vi "CS_schleife_init.vi"   [LabVIEW 2016]
uses:
  Global/Global Variables/global.vi
  Global/Global Variables/Data_Display_global.vi
  Instrument_Setup.vi
  Monitors/Utility/Monitor Communication/sub-vis/16T_Split_Cluster.vi
  Monitors/Utility/Monitor Communication/sub-vis/20T_Split_Cluster.vi
  Monitors/Utility/Monitor Communication/sub-vis/SR830_Open_Queue.vi
  Monitors/Utility/Monitor Communication/sub-vis/16T_Queue_Commands.vi
  Monitors/Utility/Monitor Communication/sub-vis/20T_Open_Queue.vi
  Monitors/Utility/Monitor Communication/sub-vis/20T_Queue_Commands.vi
types:
  T1 = typedef "16T-Cluster.ctl" = cluster{"Clamp":bool, "Switch Heater":bool, "Go to Zero":bool, "Go to set":bool, "Go to Hold":bool, "Clamped":bool, "Quenched":bool, "Rate limit":bool, "Persistent":bool, "Hold":bool, "Set":bool, "Zero":bool, "Magnet (T)":dbl, "Leads (T)":dbl, "Magnet T (K)":dbl, "Switch":bool, "Setpoint (T)":dbl, "Rate (T/min)":dbl, "Select":bool, "Sweeping":bool}
  T2 = typedef "16T_Control.ctl" = cluster{"Clamp":bool, "Switch Heater":bool, "Go to Zero":bool, "Go to Set":bool, "Go to Hold":bool, "Setpoint (T)":dbl, "Rate (T/min)":dbl, "Set Rate":bool}
  T3 = typedef "20T_Cluster.ctl" = cluster{"Clamp":bool, "Switch Heater":bool, "Go to Zero":bool, "Go to set":bool, "Go to Hold":bool, "Clamped":bool, "Quenched":bool, "Rate limit":bool, "Persistent":bool, "Hold":bool, "Set":bool, "Zero":bool, "Magnet (T)":dbl, "Leads (T)":dbl, "Magnet T (K)":dbl, "Switch":bool, "Target (T)":dbl, "Setpoint (T)":dbl, "Rate (T/min)":dbl, "Switch Heater 2":bool, "Set Rate":bool}
  T4 = typedef "20T_Control.ctl" = cluster{"Clamp":bool, "Switch Heater":bool, "Go to Zero":bool, "Go to Set":bool, "Go to Hold":bool, "Setpoint (T)":dbl, "Rate (T/min)":dbl, "Set Rate":bool}
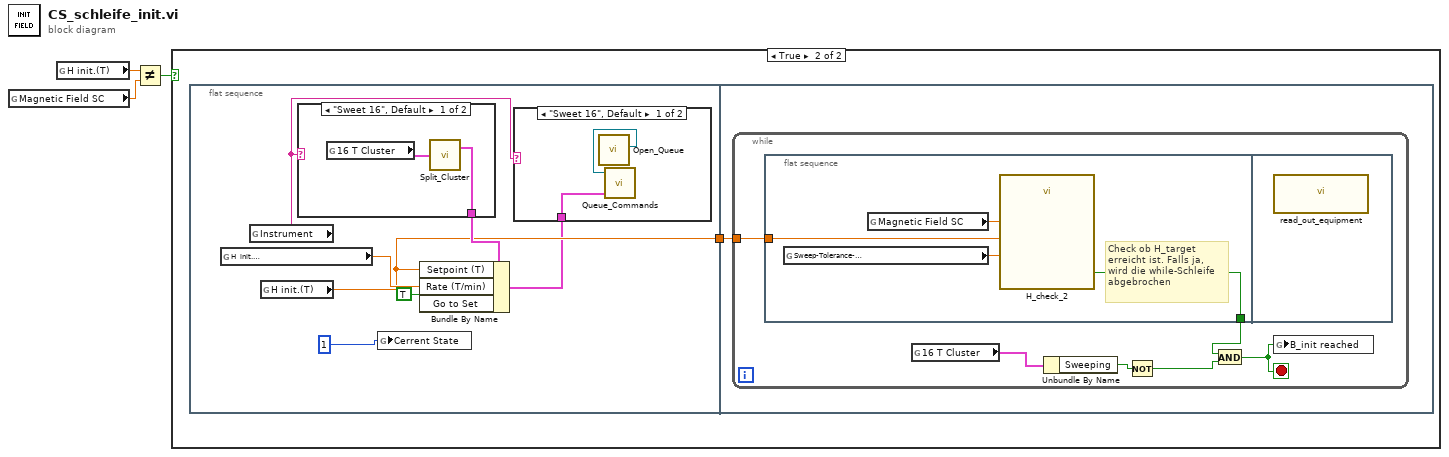
[diagram p0: block diagram]
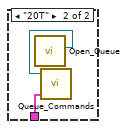
[diagram p3: hidden frame]
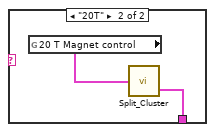
[diagram p4: hidden frame]
diagram:
  n1 = global read "Data_Display_global.vi" "Magnetic Field SC"() -> (w2:dbl)
  n2 = global read "global.vi" "H init.(T)"() -> (w3:dbl)
  n3 = Not Equal?(x=w3, y=w2) -> (x != y?=w1:bool)
  n4 = case shown="True" w1 {
    frame False {
    }
    frame True {
      n5 = flat-sequence {
        tunnel: [w8] -> w4
        tunnel: w4 -> [w20]
        frame #0 {
          n6 = global read "global.vi" "H  init. \nGeschw.(T/min)"() -> (w10:dbl)
          n7 = global read "Instrument_Setup.vi" "Instrument"() -> (w6:string)
          n8 = global read "global.vi" "H init.(T)"() -> (w8:dbl)
          n9 = case shown="\"Sweet 16\", Default" w6 {
            tunnel: [w16 w18] -> w11
            frame "Sweet 16", Default {
              n10 = global read "Data_Display_global.vi" "16 T Cluster"() -> (w17:T1)
              n11 = call-poly "Split_Cluster.vi"("16 T Magnet control"=w17) -> ("16 T Magnet control"=w16:T2)  [unwired: 1 out]
            }
            frame "20T" {
              n12 = global read "Data_Display_global.vi" "20 T Magnet control"() -> (w19:T3)
              n13 = call-poly "Split_Cluster.vi"("20 T Cluster"=w19) -> ("20 T Control"=w18:T4)  [unwired: 1 out]
            }
          }
          n14 = global write "global.vi" "Cerrent State"(1) -> ()
          n15 = Bundle By Name(cluster=w11, "Setpoint (T)"=w8, "Rate (T/min)"=w10, "Go to Set"=TRUE) -> (w5:T4)
          n16 = case shown="\"Sweet 16\", Default" w6 {
            tunnel: w5 -> [w13 w14]
            frame "Sweet 16", Default {
              n17 = call-poly "Open_Queue.vi"() -> ("queue out"=w12:refnum<queue>)  [unwired: 10 in, 1 out]
              n18 = call-poly "Queue_Commands.vi"("16 T Magnet control"=w13, "16T Queue"=w12) -> ()  [unwired: 1 in, 1 out]
            }
            frame "20T" {
              n19 = call-poly "Open_Queue.vi"() -> ("queue out"=w15:refnum<queue>)  [unwired: 10 in, 1 out]
              n20 = call-poly "Queue_Commands.vi"("20 T Control"=w14, "20T Queue"=w15) -> ()  [unwired: 1 in, 1 out]
            }
          }
        }
        frame #1 {
          n21 = while {
            tunnel: w20 -> [w26]
            stop <- w21 stop-if-true
            n22 = flat-sequence {
              tunnel: [w30] -> w23
              tunnel: w26 -> [w27]
              frame #0 {
                # "Check ob H_target\nerreicht ist. Falls ja,\nwird die while-Schleife\nabgebrochen"
                n23 = global read "Instrument_Setup.vi" "Sweep-Tolerance-\nMagnetic-Field"() -> (w29:dbl)
                n24 = global read "Data_Display_global.vi" "Magnetic Field SC"() -> (w28:dbl)
                n25 = call "H_check_2.vi"("Sweep\nTolerance %"=w29, "H_in"=w28, "H_target (K)"=w27) -> ("= H target"=w30:bool)  [unwired: 8 in]
              }
              frame #1 {
                n26 = call "read_out_equipment.vi"() -> ()  [unwired: 1 in]
              }
            }
            n27 = global read "Data_Display_global.vi" "16 T Cluster"() -> (w25:T1)
            n28 = Unbundle By Name(w25) -> ("Sweeping"=w24:bool)
            n29 = Not(x=w24) -> (.not. x?=w22:bool)
            n30 = And(x=w23, y=w22) -> (x .and. y?=w21:bool)
            n31 = global write "Data_Display_global.vi" "B_init reached"(w21) -> ()
          }
        }
      }
    }
  }
